vi "HXG2programmerFGV.vi"(5 "References in":T1, 6 "Path to Profile":path, 7 "Programmer Ctrl":T6=enum."Write Selec", 8 "error in (no error)":errorcluster, 9 "User Selections In":T2={"Run Prog"=FALSE, "Done Stop"=FALSE, "Load Profile"=FALSE, "Save Profile"=FALSE, "Repeat Execution:"=1, "Start Programmer"=FALSE, "Stop Programmer"=FALSE}, 10 "Step Array":T3[](array[typedef]), 11 "Profile Name":string) -> (0 "error out":errorcluster, 1 "References Out":T1, 2 "User Selections Out":T2={"Run Prog"=FALSE, "Done Stop"=FALSE, "Load Profile"=FALSE, "Save Profile"=FALSE, "Repeat Execution:"=1, "Start Programmer"=FALSE, "Stop Programmer"=FALSE}, 3 "Programmer Parameters":T5, 4 "Path to Profile Out":path)   [LabVIEW 2012]
uses:
  HXG2programmer.ctl
  Data Types/Programmer Step.ctl
  Data Types/Programmer Step References.ctl
  HXG2programmerUserSelections.ctl
  HXG2_ProgRefs.ctl
  <vilib>/Utility/file.llb/Read From Spreadsheet File (string).vi
  <vilib>/Utility/file.llb/Write To Spreadsheet File (string).vi
panel:
  out "Array":string[](array[string])
  out "Path to o/write":path
  out "selected path":path
  out "Path to Profile 1":path
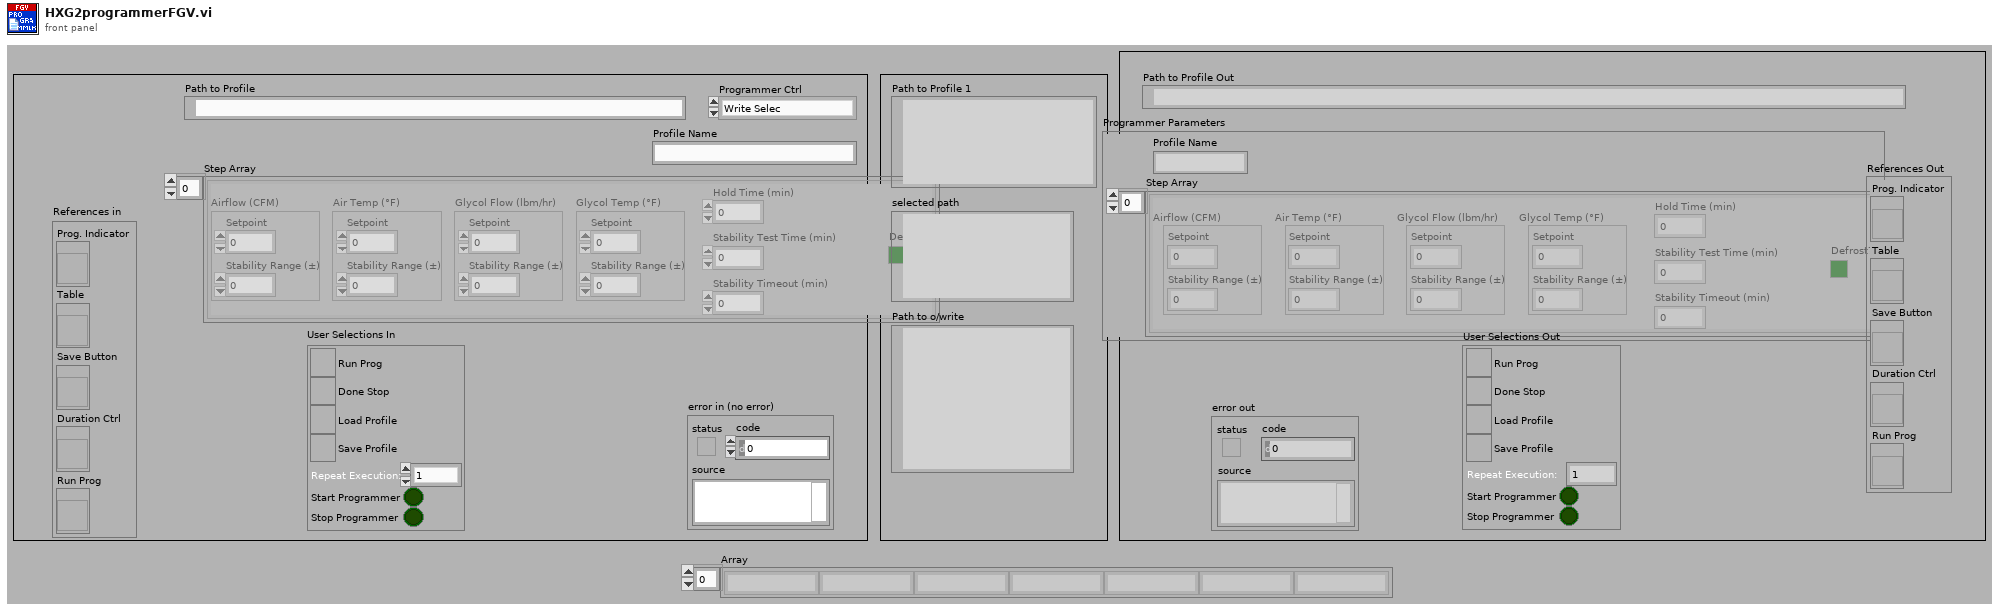
[diagram p1: front panel]
types:
  T1 = typedef "HXG2_ProgRefs.ctl" = cluster{"Prog. Indicator":refnum<vi>, "Table":refnum<vi>, "Save Button":refnum<vi>, "Duration Ctrl":refnum<vi>, "Run Prog":refnum<vi>}
  T2 = typedef "HXG2programmerUserSelections.ctl" = cluster{"Run Prog":bool, "Done Stop":bool, "Load Profile":bool, "Save Profile":bool, "Repeat Execution:":i32, "Start Programmer":bool, "Stop Programmer":bool}
  T3 = typedef "Programmer Step.ctl" = cluster{"Airflow (CFM)":T4, "Air Temp (°F)":T4, "Glycol Flow (lbm/hr)":T4, "Glycol Temp (°F)":T4, "Hold Time (min)":dbl, "Stability Test Time (min)":dbl, "Stability Timeout (min)":dbl, "Defrost?":bool}
  T4 = typedef "Programmer Step References.ctl" = cluster{"Setpoint":dbl, "Stability Range (±)":dbl}
  T5 = cluster{"Profile Name":string, "Step Array":T3[]}
  T6 = typedef "HXG2programmer.ctl" = enum16{"Write Refs", "Write Selec", "Write All", "Pass All", "React", "Write Path"}
  T7 = enum16{"Load Profile", "Save Profile", "Do Nothing"}
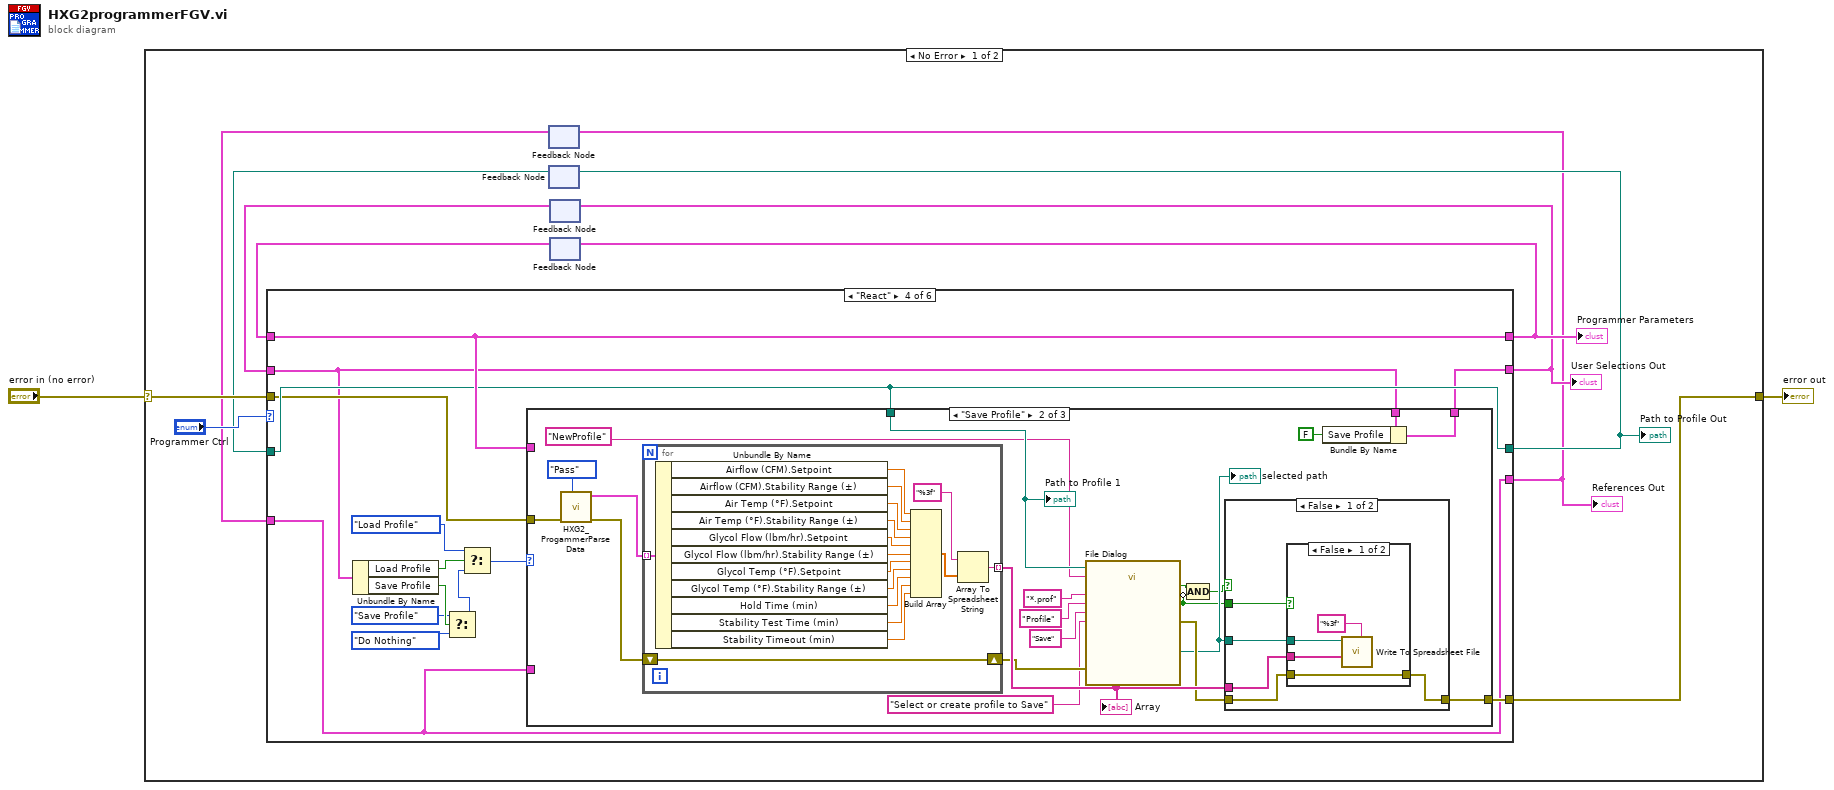
[diagram p0: block diagram]
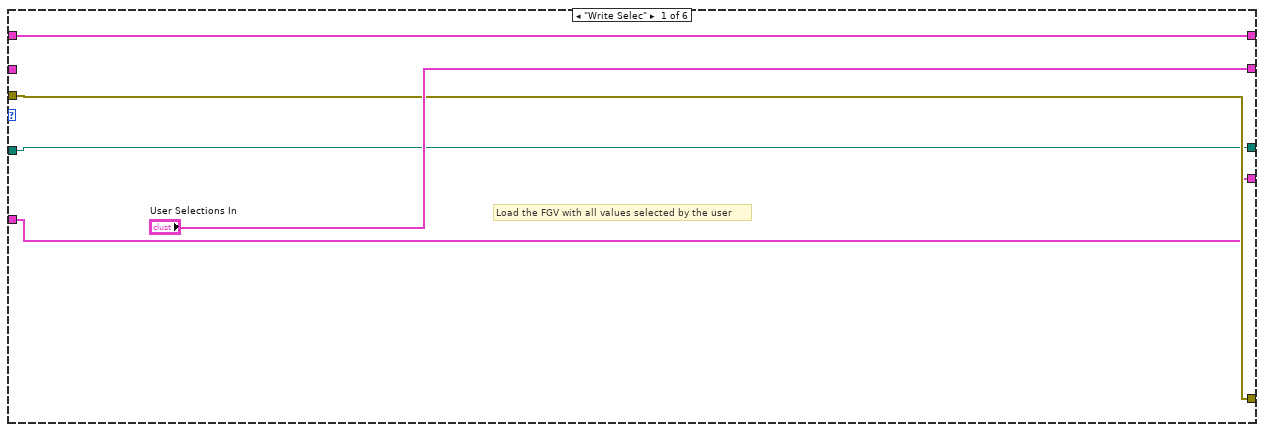
[diagram p2: hidden frame]
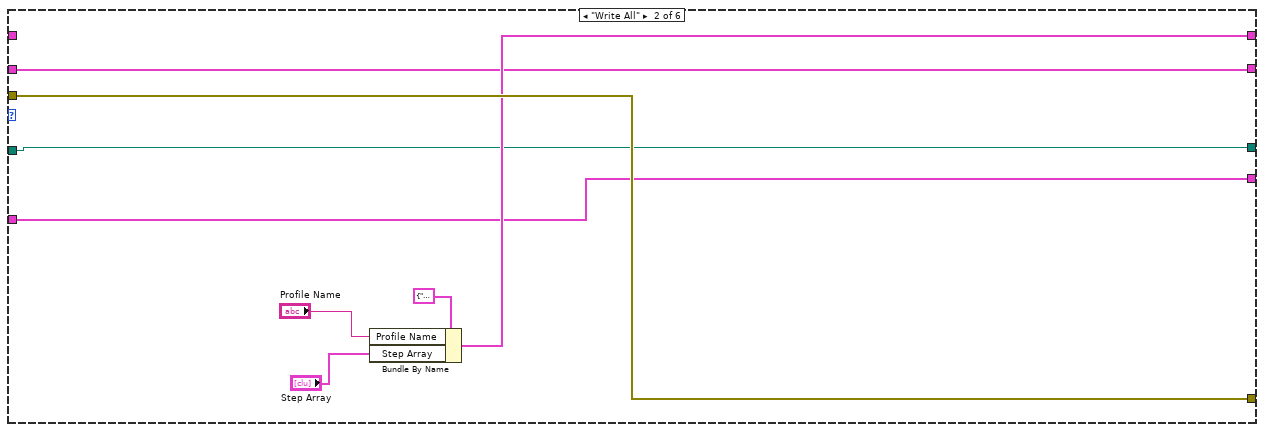
[diagram p3: hidden frame]
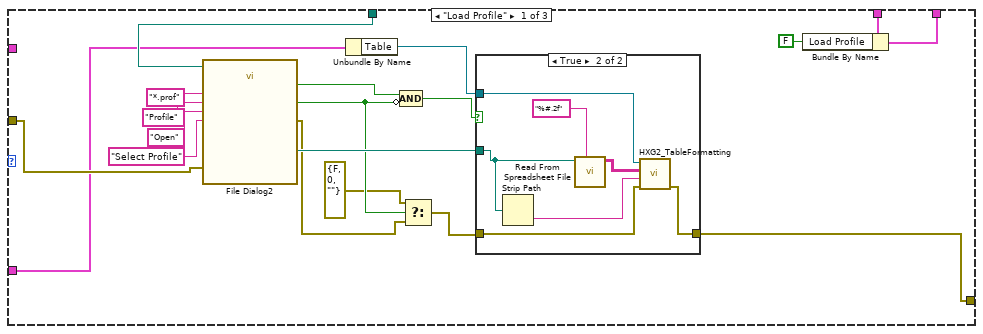
[diagram p5: hidden frame]
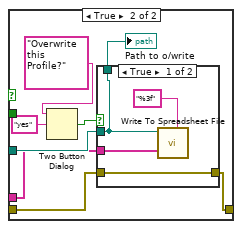
[diagram p8: hidden frame]
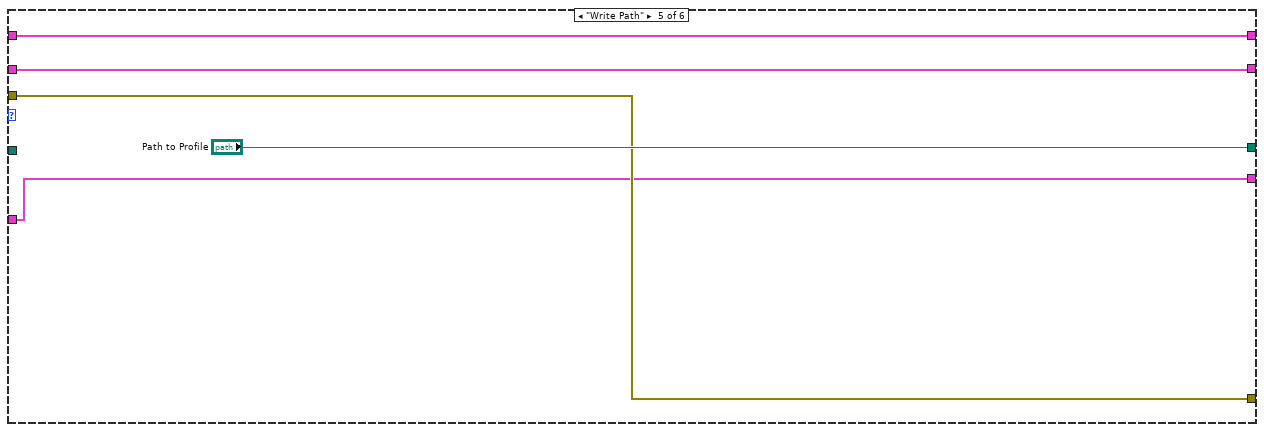
[diagram p11: hidden frame]
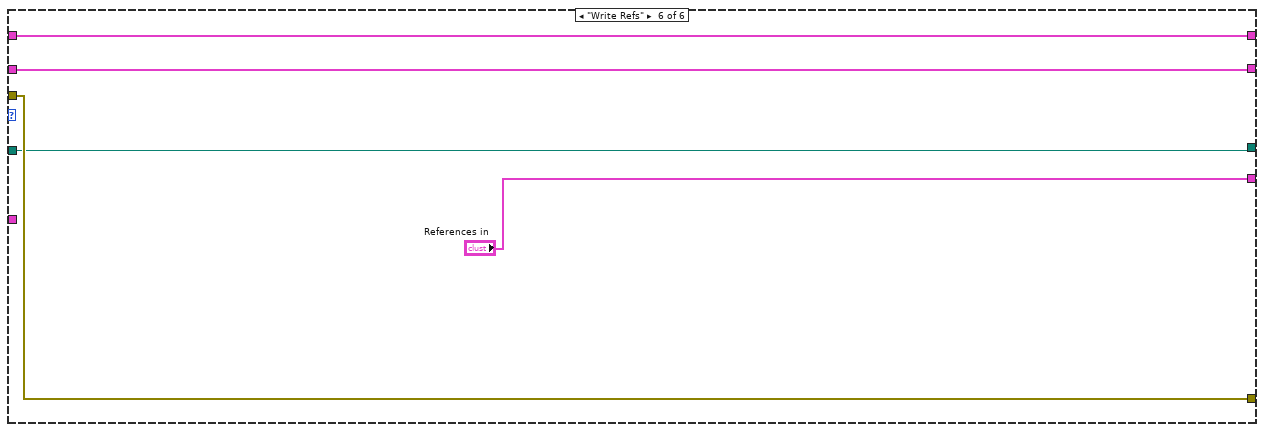
[diagram p12: hidden frame]
diagram:
  n1 = case shown="No Error" "error in (no error)" {
    selector: "error in (no error)" -> [w13 w146]
    tunnel: [w12 w146] -> w1
    frame No Error {
      n2 = feedback #1() -> (w3:T1)  [unwired: 1 in]
      n3 = feedback #2() -> (w5:path)  [unwired: 1 in]
      n4 = feedback #3() -> (w7:T2)  [unwired: 1 in]
      n5 = feedback #4() -> (w10:T5)  [unwired: 1 in]
      n6 = case shown="\"React\"" "Programmer Ctrl" {
        tunnel: w13 -> [w16 w26 w30 w36 w139 w145]
        tunnel: [w16 w26 w30 w35 w139 w145] -> w12
        tunnel: [w17 w24 w31 w38 w137 w144] -> w11
        tunnel: w10 -> [w17 _ w31 w38 w137 w144]
        tunnel: ["User Selections In" w21 w29 w33 w138 w143] -> w8
        tunnel: w7 -> [_ w21 w29 w34 w138 w143]
        tunnel: [w15 w20 w28 w37 "Path to Profile" w142] -> w6
        tunnel: w5 -> [w15 w20 w28 w37 _ w142]
        tunnel: [w14 w19 w27 w32 w136 "References in"] -> w4
        tunnel: w3 -> [w14 w19 w27 w32 w136 _]
        frame "Write Selec" {
          # "Load the FGV with all values selected by the user"
        }
        frame "Write All" {
          n7 = Bundle By Name(cluster=T5 {"Profile Name"="", "Step Array"=[{"Airflow (CFM)"={"Setpoint"=0.0, "Stability Range (±)"=0.0}, "Air Temp (°F)"={"Setpoint"=0.0, "Stability Range (±)"=0.0}, "Glycol Flow (lbm/hr)"={"Setpoint"=0.0, "Stability Range (±)"=0.0}, "Glycol Temp (°F)"={"Setpoint"=0.0, "Stability Range (±)"=0.0}, "Hold Time (min)"=0.0, "Stability Test Time (min)"=0.0, "Stability Timeout (min)"=0.0, "Defrost?"=FALSE}]} ("Programmer Parameters"), "Profile Name"="Profile Name", "Step Array"="Step Array") -> (w24:T5)
        }
        frame "Pass All" {
        }
        frame "React" {
          n8 = Unbundle By Name(w34) -> ("Load Profile"=w45:bool, "Save Profile"=w43:bool)
          n9 = Select(t=T7."Save Profile", s=w43, f=T7."Do Nothing" ("t")) -> (s? t:f=w41:T7)
          n10 = Select(t=T7."Load Profile", s=w45, f=w41) -> (s? t:f=w39:T7)
          n11 = case shown="\"Save Profile\"" w39 {
            tunnel: w38 -> [_ _ _]
            tunnel: w37 -> [w61 w91 _]
            tunnel: w36 -> [w60 w80 w135]
            tunnel: [w57 w85 w135] -> w35
            tunnel: w34 -> [w56 w83 w134]
            tunnel: [w54 w81 w134] -> w33
            tunnel: w32 -> [w53 _ _]
            frame "Load Profile" {
              n12 = call "File Dialog2"("start path"=w61, "prompt"="Select Profile" ("button label"), "button label"="Open", "error in"=w60, "pattern (all files)"="*.prof", "pattern label"="Profile" ("pattern (all files)")) -> ("selected path"=w58:path, "exists"=w51:bool, "cancelled"=w49:bool, "error out"=w48:errorcluster)  [unwired: 6 in]
              n13 = Unbundle By Name(w53) -> ("Table"=w52:refnum<vi>)
              n14 = Compound Arithmetic op=AND(w51, invert w49) -> (w50:bool)
              n15 = Select(t=errorcluster {"status"=FALSE, "code"=0, "source"=""} ("s? t:f"), s=w49, f=w48) -> (s? t:f=w47:errorcluster)
              n16 = case shown="True" w50 {
                tunnel: w47 -> [w65 w70]
                tunnel: [w65 w69] -> w57
                tunnel: w58 -> [_ w68]
                tunnel: w52 -> [_ w66]
                frame False {
                }
                frame True {
                  n17 = Strip Path(path=w68) -> (name=w67:string)  [unwired: 1 out]
                  n18 = call-poly <vilib>:"Read From Spreadsheet File.vi"("format (%s)"="%#.2f", "file path (dialog if empty)"=w68) -> ("all rows"=w71:string[][])  [unwired: 5 in, 4 out]
                  n19 = call "HXG2_TableFormatting.vi"("error IO"=w70, "Programmer File"=w67, "Data Array In"=w71, "Table Control"=w66) -> ("error out"=w69:errorcluster)  [unwired: 6 in, 1 out]
                }
              }
              n20 = Bundle By Name(cluster=w56, "Load Profile"=FALSE) -> (w54:T2)
            }
            frame "Save Profile" {
              n21 = call "HXG2_ProgammerParseData.vi"("Parse Ctrl"=enum16{"Write", "Pass"}."Pass", "error in (no error)"=w80) -> ("error out"=w79:errorcluster, "Step Array Out"=w78:T3[])  [unwired: 8 in]
              n22 = for {
                tunnel: w78 -> [w133] mode=indexing
                tunnel: [w120] -> w93 mode=indexing
                shift-right: [w118] -> w92
                shift-left: w79 -> [w118]
                n23 = Unbundle By Name(w133) -> ("Airflow (CFM).Setpoint"=w132:dbl, "Airflow (CFM).Stability Range (±)"=w131:dbl, "Air Temp (°F).Setpoint"=w130:dbl, "Air Temp (°F).Stability Range (±)"=w129:dbl, "Glycol Flow (lbm/hr).Setpoint"=w128:dbl, "Glycol Flow (lbm/hr).Stability Range (±)"=w127:dbl, "Glycol Temp (°F).Setpoint"=w126:dbl, "Glycol Temp (°F).Stability Range (±)"=w125:dbl, "Hold Time (min)"=w124:dbl, "Stability Test Time (min)"=w123:dbl, "Stability Timeout (min)"=w122:dbl)
                n24 = Build Array(w132, w131, w130, w129, w128, w127, w126, w125, w124, w123, w122) -> (w121:dbl[])
                n25 = Array To Spreadsheet String(array=w121, 3:"%3f" ("format string")) -> (spreadsheet string=w120:string)  [unwired: 1 in]
              }
              "Array" <- w93
              n26 = call "File Dialog"("start path"=w91, "prompt"="Select or create profile to Save" ("button label"), "button label"="Save", "default name"="NewProfile", "error in"=w92, "pattern (all files)"="*.prof", "pattern label"="Profile" ("pattern (all files)")) -> ("selected path"=w84:path, "exists"=w75:bool, "cancelled"=w73:bool, "error out"=w86:errorcluster)  [unwired: 5 in]
              "selected path" <- w84
              n27 = Compound Arithmetic op=AND(w75, invert w73) -> (w74:bool)
              n28 = case shown="False" w74 {
                tunnel: w93 -> [w98 w108]
                tunnel: w84 -> [w97 w109]
                tunnel: w86 -> [w95 w107]
                tunnel: [w94 w106] -> w85
                tunnel: w73 -> [w96 _]
                frame False {
                  n29 = case shown="False" w96 {
                    tunnel: w98 -> [w102 _]
                    tunnel: w97 -> [w100 _]
                    tunnel: w95 -> [w99 w103]
                    tunnel: [w99 w103] -> w94
                    frame False {
                      n30 = call-poly <vilib>:"Write To Spreadsheet File.vi"("format (%s)"="%3f", "1D data"=w102, "file path (dialog if empty)"=w100) -> ()  [unwired: 5 in, 1 out]
                    }
                    frame True {
                    }
                  }
                }
                frame True {
                  n31 = Two Button Dialog(message="Overwrite this Profile?" ("Window Title (\"\")"), 2:"yes" ("T button name (\"OK\")")) -> (T button?=w110:bool)  [unwired: 1 in]
                  n32 = case shown="True" w110 {
                    tunnel: w109 -> [w112 w116]
                    tunnel: w108 -> [w114 _]
                    tunnel: w107 -> [w113 w117]
                    tunnel: [w113 w117] -> w106
                    tunnel: [w112 w116] -> w104
                    frame True {
                      n33 = call-poly <vilib>:"Write To Spreadsheet File.vi"("format (%s)"="%3f", "1D data"=w114, "file path (dialog if empty)"=w112) -> ()  [unwired: 5 in, 1 out]
                    }
                    frame False {
                    }
                  }
                  "Path to o/write" <- w104
                }
              }
              n34 = Bundle By Name(cluster=w83, "Save Profile"=FALSE) -> (w81:T2)
              "Path to Profile 1" <- w91
            }
            frame "Do Nothing", Default {
            }
          }
        }
        frame "Write Path" {
        }
        frame "Write Refs" {
        }
      }
      "Programmer Parameters" <- w11
      "User Selections Out" <- w8
      "Path to Profile Out" <- w6
      "References Out" <- w4
      n35 = feedback-in #1(w4) -> ()
      n36 = feedback-in #2(w6) -> ()
      n37 = feedback-in #3(w8) -> ()
      n38 = feedback-in #4(w11) -> ()
    }
    frame Error {
    }
  }
  "error out" <- w1
